vi "Normalize Coordinates2.vi"(9 "Camera Type":T1, 10 "Targets":T4(array[cluster]), 11 "Image in":T5) -> (2 "Found Totes":T2(array[cluster]) {"Normalized Rect"."Numeric 5" format="%#_2g"; "Normalized Rect"."Numeric 3" format="%#_2g"; "Normalized Rect"."Numeric 2" format="%#_2g"; "Normalized Rect"."Numeric" format="%#_2g"}, 3 "Sorted Scores":T3(array[cluster]) {"Correlation" format="%#_3g"; "Scale" format="%#_3g"; "Score" format="%#_3g"})   [LabVIEW 2014]
doc: "Normalize the rectangle and center so that they range from -1 to 1, left to right and bottom to top. This helps with producing joystick coordinates for driving the robot."
uses:
  <vilib>/vision/Image Controls.llb/IMAQ Image.ctl
  Program Files (x86)/National Instruments/LabVIEW 2014/examples/FRC/roboRIO/Vision/2015 Vision Example/Vision Support Code/Camera Types.ctl
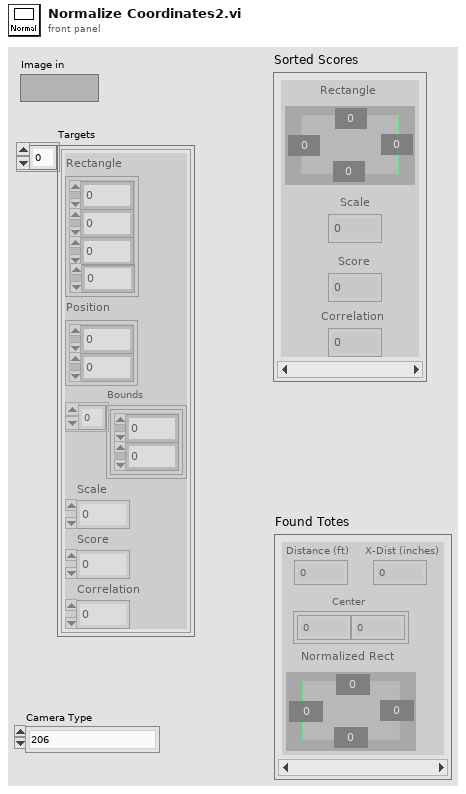
[diagram p1: front panel]
types:
  T1 = typedef "Camera Types.ctl" = enum16{"206", "1011", "1013", "MS HD3000 square", "MS HD3000 640x480"}
  T2 = cluster{"Distance (ft)":dbl, "X-Dist (inches)":dbl, "Center":cluster{dbl, dbl}, "Normalized Rect":cluster{"Numeric":dbl, "Numeric 2":dbl, "Numeric 3":dbl, "Numeric 5":dbl}}[]
  T3 = cluster{"Rectangle":cluster{"Numeric":dbl, "Numeric 2":dbl, "Numeric 3":dbl, "Numeric 5":dbl}, "Scale":dbl, "Score":dbl, "Correlation":dbl}[]
  T4 = cluster{"Rectangle":cluster{"Numeric":dbl, "Numeric 2":dbl, "Numeric 3":dbl, "Numeric 5":dbl}, "Position":cluster{"Numeric":dbl, "Numeric 2":dbl}, "Bounds":cluster{"Numeric":dbl, "Numeric 2":dbl}[], "Scale":dbl, "Score":dbl, "Correlation":dbl}[]
  T5 = typedef "IMAQ Image.ctl" = refnum<image>
  T6 = cluster{"X Resolution":i32, i32, "X Resolution":i32, i32}
  T7 = cluster{"[0]":dbl, "[1]":dbl, "[2]":dbl, "[3]":dbl}
  T8 = cluster{"Numeric":dbl, "Numeric 2":dbl, "Numeric 3":dbl, "Numeric 5":dbl}
  T9 = cluster{"Rectangle":cluster{"Numeric":dbl, "Numeric 2":dbl, "Numeric 3":dbl, "Numeric 5":dbl}, "Scale":dbl, dbl, dbl}
  T10 = cluster{"Distance (ft)":dbl, dbl, cluster{dbl, dbl}, cluster{dbl, dbl, dbl, dbl}}
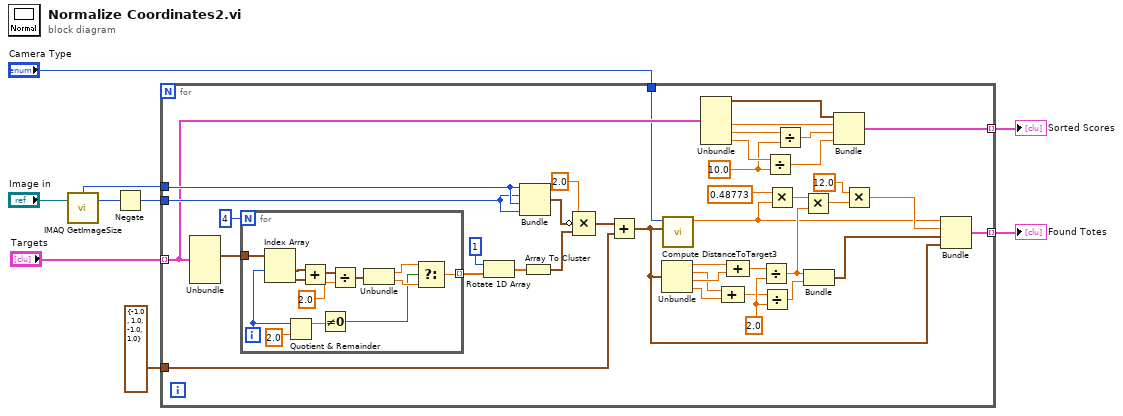
[diagram p0: block diagram]
diagram:
  n1 = call "IMAQ GetImageSize"("Image"="Image in") -> ("Y Resolution"=w7:i32, "X Resolution"=w8:i32)  [unwired: 3 in, 1 out]
  n2 = Negate(x=w7) -> (-x=w9:i32)
  n3 = for {
    tunnel: "Targets" -> [w33] mode=indexing
    tunnel: w9 -> [w48]
    tunnel: w8 -> [w49]
    tunnel: [w36] -> w4 mode=indexing
    tunnel: [w30] -> w1 mode=indexing
    tunnel: cluster{dbl, dbl, dbl, dbl} {-1.0, 1.0, -1.0, 1.0} ("y") -> [w34]
    tunnel: "Camera Type" -> [w24]
    w25 = 10.0
    w40 = 2.0
    n4 = Unbundle(w33) -> ("Bounds"=w22:cluster{"Numeric":dbl, "Numeric 2":dbl}[])  [unwired: 5 out]
    n5 = for {
      N: 4 -> [_]
      tunnel: w22 -> [w62]
      tunnel: [w50] -> w18 mode=indexing
      i -> [w54]
      n6 = Index Array(array=w62, index #1=w54) -> (element #1=w61:cluster{"Numeric":dbl, "Numeric 2":dbl}, element #2=w60:cluster{"Numeric":dbl, "Numeric 2":dbl})  [unwired: 1 in]
      n7 = Quotient & Remainder(x=w54, y=2.0) -> (x-y*floor(x/y)=w52:dbl)  [unwired: 1 out]
      n8 = Add(x=w61, y=w60) -> (x+y=w59:cluster{"Numeric":dbl, "Numeric 2":dbl})
      n9 = Not Equal To 0?(x=w52) -> (x != 0?=w51:bool)
      n10 = Divide(x=w59, y=2.0) -> (x/y=w57:cluster{"Numeric":dbl, "Numeric 2":dbl})
      n11 = Unbundle(w57) -> ("Numeric"=w56:dbl, "Numeric 2"=w55:dbl)
      n12 = Select(t=w56, s=w51, f=w55) -> (s? t:f=w50:dbl)
    }
    n13 = Rotate 1D Array(1:w18, 2:1) -> (0:w19:dbl[])
    n14 = Bundle("X Resolution"=w49, w48, "X Resolution"=w49, w48) -> (w47:T6)  [unwired: 1 in]
    n15 = Array To Cluster(array=w19) -> (cluster=w20:T7)
    n16 = Compound Arithmetic op=MULTIPLY(2.0, invert w47, w20) -> (w46:cluster{dbl, dbl, dbl, dbl})
    n17 = Add(x=w46, y=w34) -> (x+y=w23:cluster{dbl, dbl, dbl, dbl})
    n18 = Unbundle(w23) -> (w44:dbl, w41:dbl, w43:dbl, w42:dbl)
    n19 = call "Compute DistanceToTarget3.vi"("Norm Rect"=w23, "Camera Type"=w24) -> ("Distance (ft)"=w10:dbl)  [unwired: 9 in]
    n20 = Unbundle(w33) -> ("Rectangle"=w31:T8, "Scale"=w32:dbl, "Score"=w26:dbl, "Correlation"=w29:dbl)  [unwired: 2 out]
    n21 = Compound Arithmetic op=ADD(w41, w42) -> (w38:dbl)
    n22 = Compound Arithmetic op=ADD(w44, w43) -> (w39:dbl)
    n23 = Divide(x=w39, y=w40) -> (x/y=w14:dbl)
    n24 = Divide(x=w38, y=w40) -> (x/y=w37:dbl)
    n25 = Divide(x=w29, y=w25) -> (x/y=w28:dbl)
    n26 = Multiply(x=0.48773 ("y"), y=w10) -> (x*y=w15:dbl)
    n27 = Divide(x=w26, y=w25) -> (x/y=w27:dbl)
    n28 = Multiply(x=w15, y=w14) -> (x*y=w13:dbl)
    n29 = Bundle(w14, w37) -> (w35:cluster{dbl, dbl})  [unwired: 1 in]
    n30 = Bundle("Rectangle"=w31, "Scale"=w32, w27, w28) -> (w30:T9)  [unwired: 1 in]
    n31 = Multiply(x=12.0, y=w13) -> (x*y=w11:dbl)
    n32 = Bundle("Distance (ft)"=w10, w11, w35, w23) -> (w36:T10)  [unwired: 1 in]
  }
  "Sorted Scores" <- w1
  "Found Totes" <- w4
